vi "rotGroupDof.vi"(7 "DOF Group":T1, 8 "error in (no error)":errorcluster, 9 "Tilt Angle (arcsec)":cluster{"Tile X":dbl, "Tilt Y":dbl}, 10 "State in DOF":dbl[](array[numeric]), 11 "CamRot in":refnum<class "CamRot.lvclass">) -> (0 "error out":errorcluster, 2 "Rotated State in DOF":dbl[](array[numeric]), 3 "CamRot out":refnum<class "CamRot.lvclass">)   [LabVIEW 2016, in "OfcFunc.lvlib" / "CamRot.lvclass"]
doc: "Rotate the degree of freedom of specific group."
uses:
  CamRot.lvclass
  StrictDef/DofGroup.ctl
  OfcFunc.lvlib
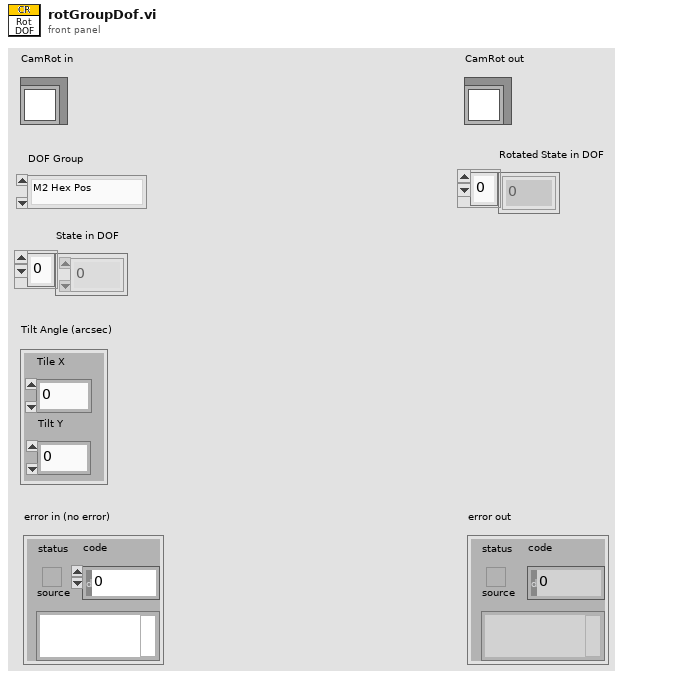
[diagram p1: front panel]
types:
  T1 = typedef "OfcFunc.lvlib/DofGroup.ctl" = enum16{"M2 Hex Pos", "Cam Hex Pos", "M1M3 Bend", "M2 Bend"}
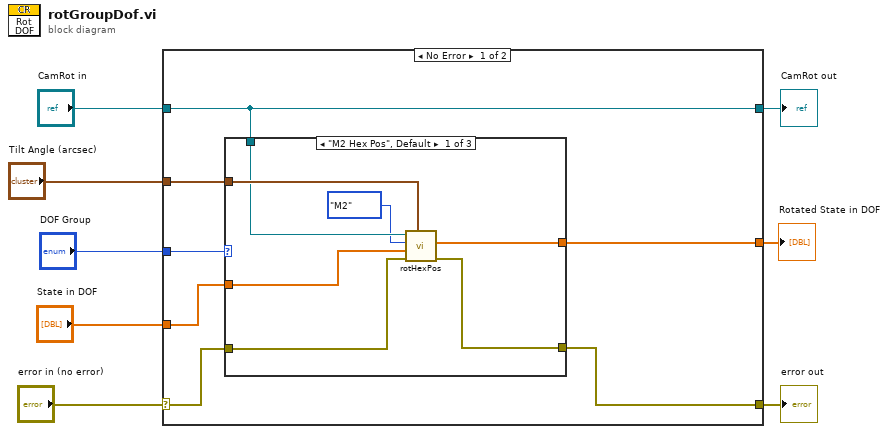
[diagram p0: block diagram]
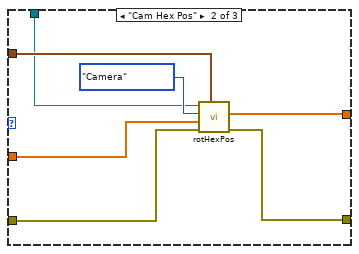
[diagram p2: hidden frame]
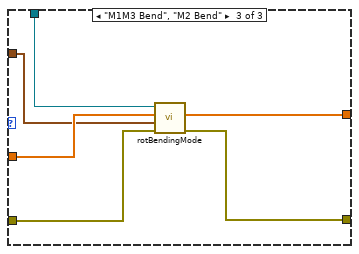
[diagram p3: hidden frame]
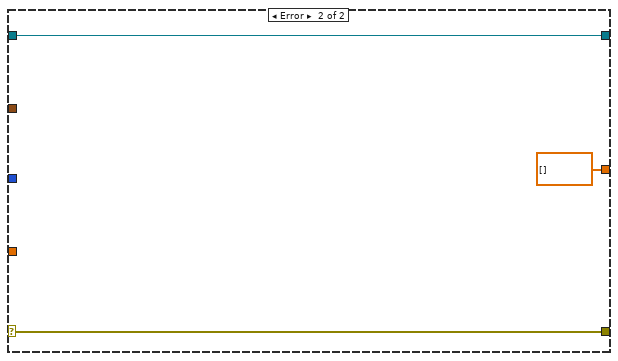
[diagram p4: hidden frame]
diagram:
  n1 = case shown="No Error" "error in (no error)" {
    selector: "error in (no error)" -> [w11 w38]
    tunnel: [w10 w38] -> w7
    tunnel: [w14 w37] -> w5
    tunnel: "CamRot in" -> [w14 w37]
    tunnel: "DOF Group" -> [w15 _]
    tunnel: "Tilt Angle (arcsec)" -> [w13 _]
    tunnel: "State in DOF" -> [w12 _]
    tunnel: [w9 dbl[] [] ("Rotated Hexapod DOF")] -> w1
    frame No Error {
      n2 = case shown="\"M2 Hex Pos\", Default" w15 {
        tunnel: w14 -> [w21 w27 w35]
        tunnel: w13 -> [w22 w28 w33]
        tunnel: w12 -> [w19 w26 w34]
        tunnel: w11 -> [w18 w25 w32]
        tunnel: [w17 w24 w31] -> w10
        tunnel: [w16 w23 w30] -> w9
        frame "M2 Hex Pos", Default {
          n3 = call "rotHexPos.vi"("Tilt Angle (arcsec)"=w22, "error in (no error)"=w18, "Hexapod DOF"=w19, "Hexapod"=enum16{"Camera", "M2"}."M2", "CamRot in"=w21) -> ("error out"=w17:errorcluster, "Rotated Hexapod DOF"=w16:dbl[])  [unwired: 4 in, 1 out]
        }
        frame "Cam Hex Pos" {
          n4 = call "rotHexPos.vi"("Tilt Angle (arcsec)"=w28, "error in (no error)"=w25, "Hexapod DOF"=w26, "Hexapod"=enum16{"Camera", "M2"}."Camera", "CamRot in"=w27) -> ("error out"=w24:errorcluster, "Rotated Hexapod DOF"=w23:dbl[])  [unwired: 4 in, 1 out]
        }
        frame "M1M3 Bend", "M2 Bend" {
          n5 = call "rotBendingMode.vi"("error in (no error)"=w32, "Tilt Angle (arcsec)"=w33, "Mirror DOF (um)"=w34, "CamRot in"=w35) -> ("error out"=w31:errorcluster, "Rotated Mirror DOF (um)"=w30:dbl[])  [unwired: 5 in, 1 out]
        }
      }
    }
    frame Error {
    }
  }
  "error out" <- w7
  "CamRot out" <- w5
  "Rotated State in DOF" <- w1
